vi "ReadFileSpectrumSimple.vi"() -> ()   [LabVIEW 2020]
panel:
  out "subarray":dbl[](array[numeric])
  out "all rows":dbl[][](array[numeric])
  in  "file path (dialog if empty)":path
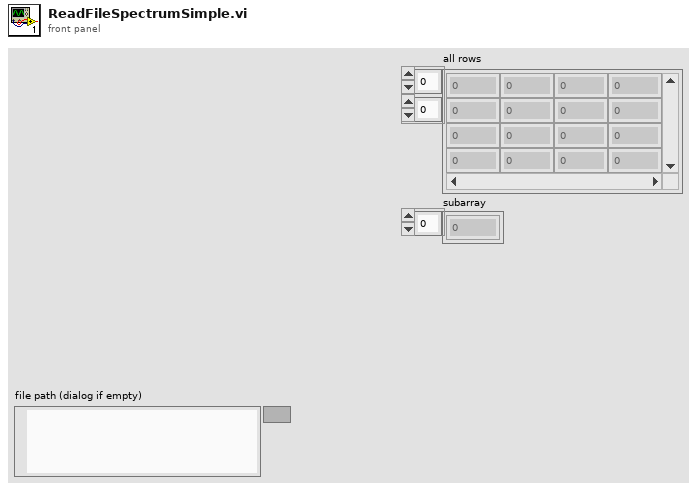
[diagram p1: front panel]
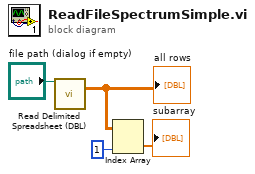
[diagram p0: block diagram]
diagram:
  n1 = call "Read Delimited Spreadsheet (DBL).vi"("file path (dialog if empty)"="file path (dialog if empty)") -> ("all rows"=w3:dbl[][])  [unwired: 9 in, 5 out]
  "all rows" <- w3
  n2 = Index Array(array=w3, index (col)=1 ("disabled index (col)")) -> (element=→"subarray":dbl[])  [unwired: 1 in]
